vi "Evaluate New Day.vi"(8 "error in (no error)":errorcluster, 11 "Text File Sink in":refnum<class "Text File Sink.lvclass">) -> (0 "error out":errorcluster, 3 "Text File Sink out":refnum<class "Text File Sink.lvclass">)   [LabVIEW 2018, in "MVA Framework.lvlib" / "Text File Sink.lvclass"]
doc: "--\nCopyright © 2017 Composed SystemsI All rights reserved.\n\nAuthor: Jon McBee <jon.mcbee@composed.io>\n\nThis library is provided \"AS IS\" ,WITHOUT WARRANTIES OR\nCONDITIONS OF ANY KIND, either express or implied.\n\nComposed Systems -- composed.io\n\nStream 0.0.1.1\nJon McBee - Composed Systems\nCopyright (c) 2017, Composed Systems"
uses:
  Text File Sink.lvclass
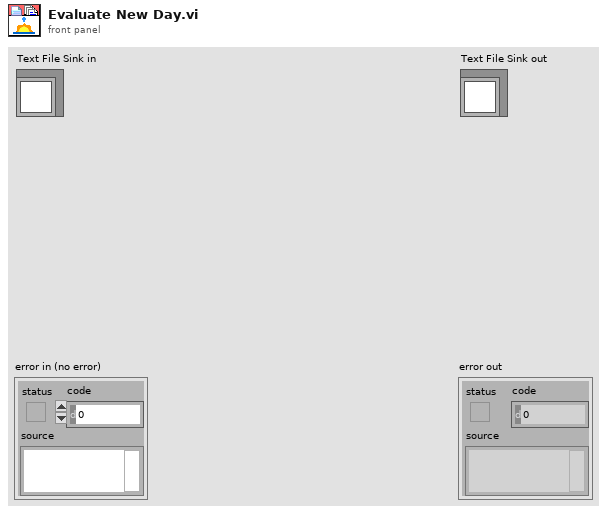
[diagram p1: front panel]
types:
  T1 = typedef "LVDateTimeRec.ctl" = cluster{"fractional second":dbl, "second":i32, "minute":i32, "hour":i32, "day of month":i32, "month":i32, "year":i32, "day of week":i32, "day of year":i32, "DST":i32}
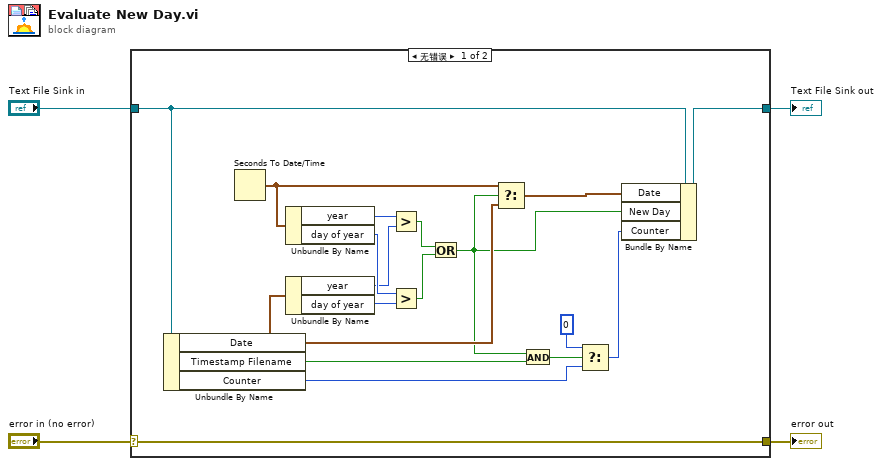
[diagram p0: block diagram]
diagram:
  n1 = case shown="无错误" "error in (no error)" {
    selector: "error in (no error)" -> [w22 w24]
    tunnel: [w22 w24] -> w3
    tunnel: [w11 w23] -> w1
    tunnel: "Text File Sink in" -> [w12 w23]
    frame No Error {
      n2 = Unbundle By Name(w12) -> ("Date"=w14:T1, "Timestamp Filename"=w8:bool, "Counter"=w7:u16)
      n3 = Seconds To Date/Time() -> (date time rec=w21:T1)  [unwired: 2 out]
      n4 = Unbundle By Name(w21) -> ("year"=w20:i32, "day of year"=w19:i32)
      n5 = Unbundle By Name(w14) -> ("year"=w17:i32, "day of year"=w18:i32)
      n6 = Greater?(x=w20, y=w17) -> (0:w15:bool)
      n7 = Greater?(x=w19, y=w18) -> (0:w16:bool)
      n8 = Or(x=w15, y=w16) -> (x .or. y?=w9:bool)
      n9 = Select(t=w21, s=w9, f=w14) -> (s? t:f=w13:T1)
      n10 = And(x=w9, y=w8) -> (x .and. y?=w10:bool)
      n11 = Select(t=u16 0, s=w10, f=w7) -> (s? t:f=w5:u16)
      n12 = Bundle By Name(cluster=w12, "Date"=w13, "New Day"=w9, "Counter"=w5) -> (w11:refnum<class "Text File Sink.lvclass">)
    }
    frame Error {
    }
  }
  "error out" <- w3
  "Text File Sink out" <- w1
